vi "Usage Nunchuk.vi"() -> ()   [LabVIEW 2011, in "Wiimote.lvlib"]
uses:
  Wiimote.lvlib
  Wiimote Buttons.ctl
  Nunchuk Buttons.ctl
panel:
  out "Nunchuk Analog Stick":cluster{"X":u16, "Y":u16}[](graph)
  out "Nunchuk Acceleration":T1(graph)
  out "Wiimote Acceleration":T1(graph)
  out "Nunchuk Buttons":T2
  in  "index":i32
  out "IR Sensor":cluster{"X":u16, "Y":u16}[](graph)
  out "Wiimote Buttons":T3
  in  "stop":bool
  out "error out":errorcluster
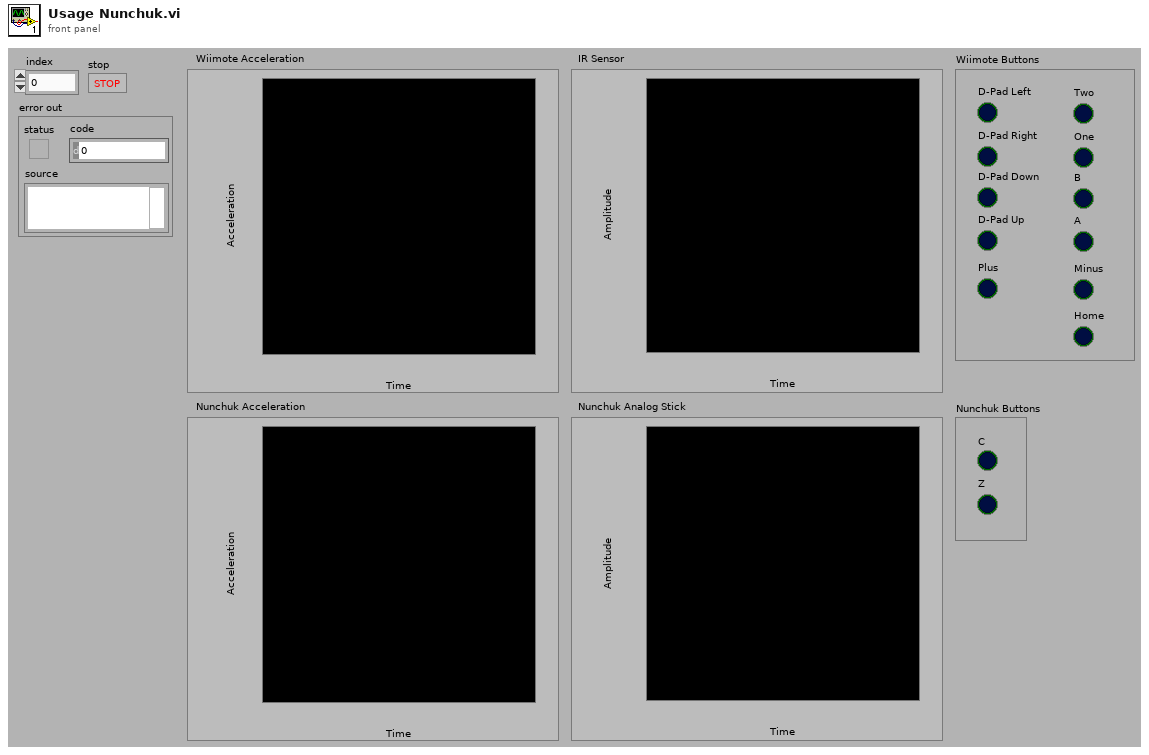
[diagram p1: front panel]
types:
  T1 = cluster{"Acceleration X":dbl, "Acceleration Y":dbl, "Acceleration Z":dbl}
  T2 = typedef "Wiimote.lvlib/Nunchuk Buttons.ctl" = cluster{"C":bool, "Z":bool}
  T3 = typedef "Wiimote.lvlib/Wiimote Buttons.ctl" = cluster{"D-Pad Left":bool, "D-Pad Right":bool, "D-Pad Down":bool, "D-Pad Up":bool, "Plus":bool, "Two":bool, "One":bool, "B":bool, "A":bool, "Minus":bool, "Home":bool}
  T4 = typedef "Wiimote.lvlib/Wiimote Acceleration.ctl" = cluster{"Acceleration X":dbl, "Acceleration Y":dbl, "Acceleration Z":dbl}
  T5 = cluster{"Wiimote 0G Calibration":T4, "Wiimote 1G Calibration":T4, "Nunchuk 0G Calibration":T4, "Nunchuk 1G Calibration":T4}
  T6 = typedef "Wiimote.lvlib/Wiimote IR Sensor.ctl" = cluster{"Point 1":T7, "Point 2":T7, "Point 3":T7, "Point 4":T7}
  T7 = typedef "Wiimote.lvlib/Wiimote Point.ctl" = cluster{"X":u16, "Y":u16}
  T8 = cluster{"Wiimote Buttons":T3, "Wiimote Acceleration Raw":T4, "Wiimote IR Sensor":T6, "Nunchuk Analog Stick":T7, "Nunchuk Acceleration Raw":T4, "Nunchuk Buttons":T2}
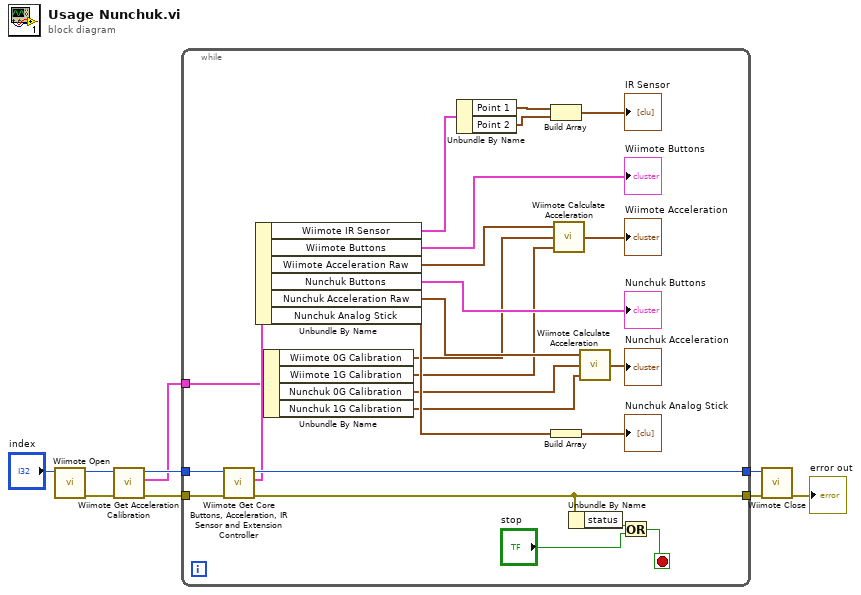
[diagram p0: block diagram]
diagram:
  n1 = call "Wiimote Open.vi"("index"="index") -> ("error out"=w3:errorcluster, "hWiimoteHandle"=w5:u32)  [unwired: 9 in]
  n2 = call "Wiimote Get Acceleration Calibration.vi"("error in"=w3, "hWiimoteHandle in"=w5) -> ("error out"=w2:errorcluster, "Calibration Data Out"=w1:T5, "hWiimoteHandle out"=w4:u32)  [unwired: 7 in]
  n3 = while {
    tunnel: w4 -> [w34]
    tunnel: w2 -> [w33]
    tunnel: [w32] -> w8
    tunnel: [w28] -> w7
    tunnel: w1 -> [w14]
    stop <- w25 stop-if-true
    n4 = call "Wiimote Get Core Buttons, Acceleration, IR Sensor and Extension Controller.vi"("error in"=w33, "hWiimoteHandle in"=w34) -> ("error out"=w28:errorcluster, "Data out"=w24:T8, "hWiimoteHandle out"=w32:u32)  [unwired: 7 in]
    n5 = Unbundle By Name(w24) -> ("Wiimote IR Sensor"=w23:T6, "Wiimote Buttons"=→"Wiimote Buttons":T3, "Wiimote Acceleration Raw"=w17:T4, "Nunchuk Buttons"=→"Nunchuk Buttons":T2, "Nunchuk Acceleration Raw"=w16:T4, "Nunchuk Analog Stick"=w20:T7)
    n6 = Unbundle By Name(w14) -> ("Wiimote 0G Calibration"=w10:T4, "Wiimote 1G Calibration"=w11:T4, "Nunchuk 0G Calibration"=w12:T4, "Nunchuk 1G Calibration"=w13:T4)
    n7 = Unbundle By Name(w23) -> ("Point 1"=w31:T7, "Point 2"=w30:T7)
    n8 = Build Array(w31, w30) -> (→"IR Sensor":T7[])
    n9 = Build Array(w20) -> (→"Nunchuk Analog Stick":T7[])
    n10 = call "Wiimote Calculate Acceleration.vi"("Acceleration 1G Calibration"=w11, "Acceleration 0G Calibration"=w10, "Acceleration Raw in"=w17) -> ("Acceleration Calibrated Out"=→"Wiimote Acceleration":T4)
    n11 = Unbundle By Name(w28) -> ("status"=w27:bool)
    n12 = call "Wiimote Calculate Acceleration.vi"("Acceleration 1G Calibration"=w13, "Acceleration 0G Calibration"=w12, "Acceleration Raw in"=w16) -> ("Acceleration Calibrated Out"=→"Nunchuk Acceleration":T4)
    n13 = Or(x=w27, y="stop") -> (x .or. y?=w25:bool)
  }
  n14 = call "Wiimote Close.vi"("error in"=w7, "hWiimoteHandle in"=w8) -> ("error out"=→"error out":errorcluster)  [unwired: 9 in]
